vi "Sol_Tierra_Luna_2.vi"() -> ()   [LabVIEW 2016]
panel:
  out "Luna":bool
  in  "Posición Horizontal":i32(slide) scale=0.0..100.0
  in  "Posición Vertical":i32(slide) scale=0.0..100.0
  in  "Stop Button":bool
  out "Tierra":bool
  out "Sol":bool
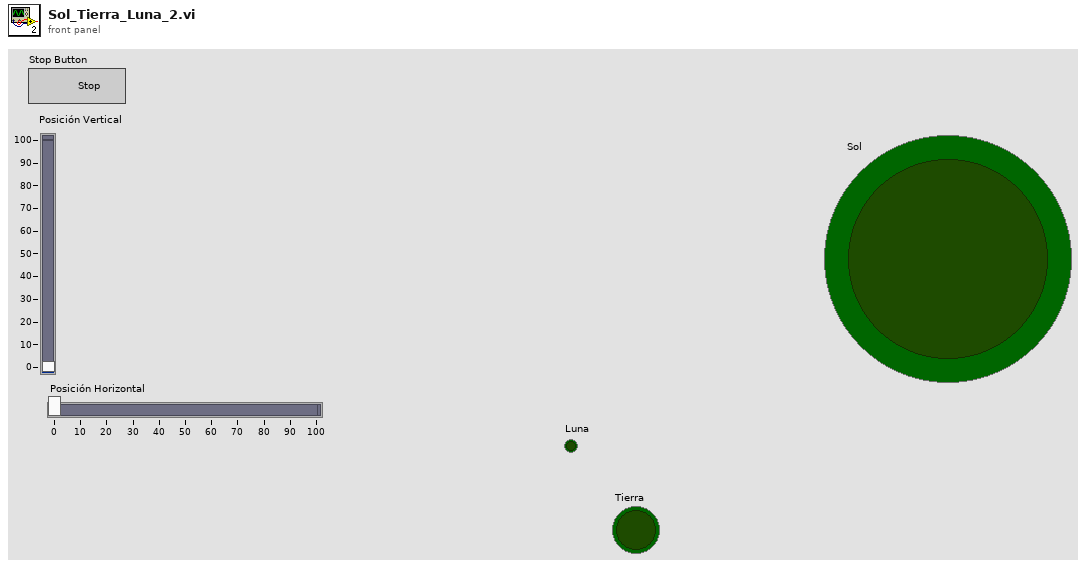
[diagram p1: front panel]
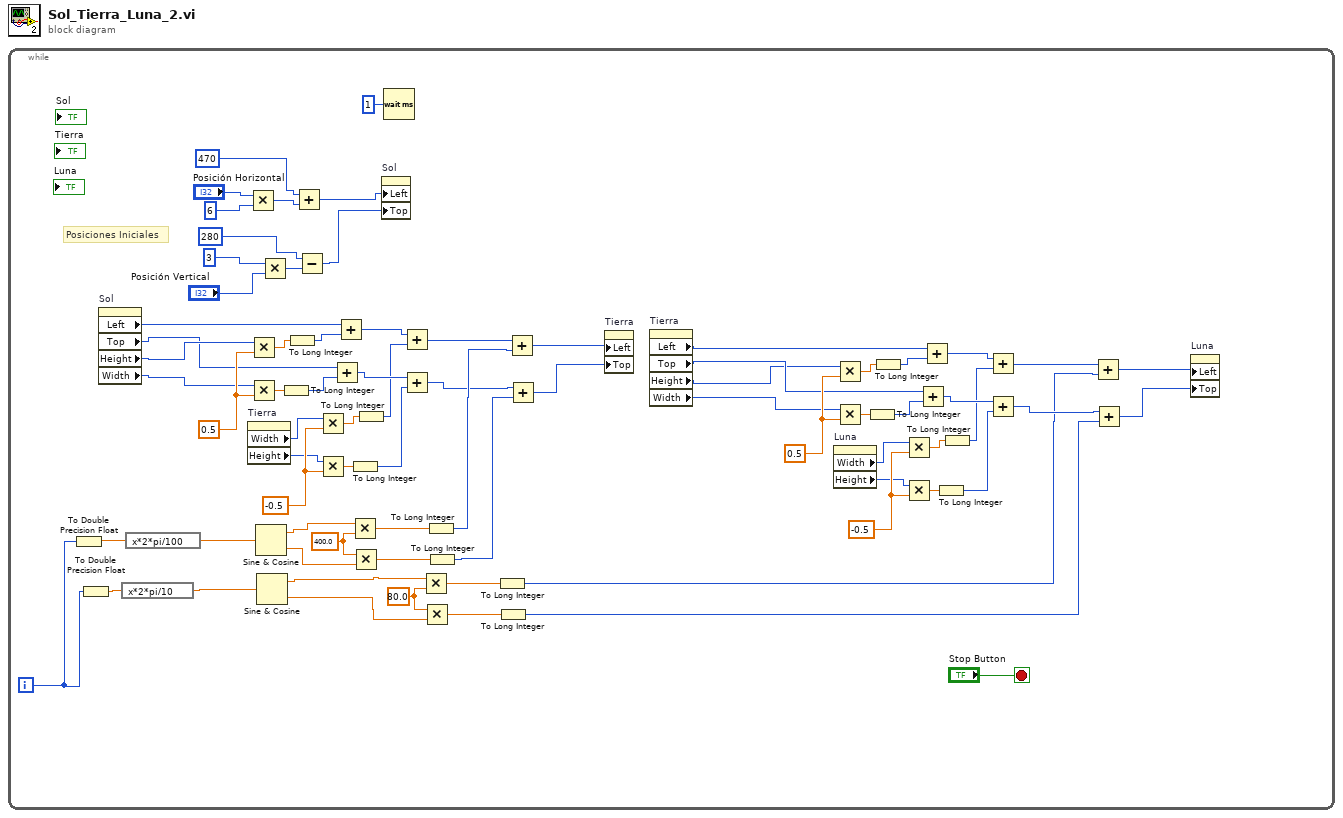
[diagram p0: block diagram]
diagram:
  n1 = while {
    i -> [w40]
    stop <- "Stop Button" stop-if-true
    w17 = -0.5 ("y")
    w20 = 0.5 ("y")
    w29 = 80.0 ("y")
    w38 = 400.0 ("y")
    w62 = -0.5 ("y")
    w69 = 0.5 ("y")
    # "Posiciones Iniciales"
    n2 = To Double Precision Float(number=w40) -> (double precision float=w41:dbl)
    n3 = To Double Precision Float(number=w40) -> (double precision float=w43:dbl)
    n4 = property on="Sol" class="Bool (strict)"() -> ("Left"=w65:i32, "Top"=w66:i32, "Height"=w67:u32, "Width"=w68:u32)  [unwired: 2 in, 2 out]
    n5 = expression code="x*2*pi/10"(w43) -> (w45:dbl)
    n6 = expression code="x*2*pi/100"(w41) -> (w44:dbl)
    n7 = Multiply(x="Posición Horizontal", y=6) -> (x*y=w48:i32)
    n8 = property on="Tierra" class="Bool (strict)"() -> ("Width"=w61:u32, "Height"=w60:u32)  [unwired: 2 in, 2 out]
    n9 = Multiply(x=w67, y=w69) -> (x*y=w71:dbl)
    n10 = Multiply(x=w68, y=w69) -> (x*y=w73:dbl)
    n11 = Sine & Cosine(0:w44) -> (1:w39:dbl, 2:w42:dbl)
    n12 = Sine & Cosine(0:w45) -> (1:w26:dbl, 2:w25:dbl)
    n13 = Multiply(x=3, y="Posición Vertical") -> (x*y=w55:i32)
    n14 = To Long Integer(number=w73) -> (32bit integer=w72:i32)
    n15 = To Long Integer(number=w71) -> (32bit integer=w70:i32)
    n16 = Add(x=470 ("Position:Left"), y=w48) -> (x+y=w47:i32)
    n17 = Subtract(x=280 ("Position:Top"), y=w55) -> (x-y=w46:i32)
    n18 = Multiply(x=w61, y=w62) -> (x*y=w63:dbl)
    n19 = Multiply(x=w60, y=w62) -> (x*y=w64:dbl)
    n20 = Add(x=w66, y=w72) -> (x+y=w59:i32)
    n21 = Add(x=w65, y=w70) -> (x+y=w58:i32)
    n22 = To Long Integer(number=w64) -> (32bit integer=w56:i32)
    n23 = Multiply(x=w39, y=w38) -> (x*y=w36:dbl)
    n24 = Multiply(x=w38, y=w42) -> (x*y=w37:dbl)
    n25 = To Long Integer(number=w63) -> (32bit integer=w57:i32)
    n26 = property on="Sol" class="Bool (strict)"("Left"=w47, "Top"=w46) -> ()  [unwired: 2 in, 2 out]
    n27 = Wait (ms)(milliseconds to wait=u32 1) -> ()  [unwired: 1 out]
    n28 = Add(x=w58, y=w57) -> (x+y=w32:i32)
    n29 = Add(x=w59, y=w56) -> (x+y=w33:i32)
    n30 = Multiply(x=w26, y=w29) -> (x*y=w27:dbl)
    n31 = Multiply(x=w29, y=w25) -> (x*y=w28:dbl)
    n32 = To Long Integer(number=w36) -> (32bit integer=w35:i32)
    n33 = To Long Integer(number=w37) -> (32bit integer=w34:i32)
    n34 = To Long Integer(number=w27) -> (32bit integer=w4:i32)
    n35 = To Long Integer(number=w28) -> (32bit integer=w3:i32)
    n36 = Add(x=w32, y=w35) -> (x+y=w31:i32)
    n37 = Add(x=w33, y=w34) -> (x+y=w30:i32)
    n38 = property on="Tierra" class="Bool (strict)"("Left"=w31, "Top"=w30) -> ()  [unwired: 2 in, 2 out]
    n39 = property on="Tierra" class="Bool (strict)"() -> ("Left"=w8:i32, "Top"=w7:i32, "Height"=w6:u32, "Width"=w5:u32)  [unwired: 2 in, 2 out]
    n40 = property on="Luna" class="Bool (strict)"() -> ("Width"=w16:u32, "Height"=w15:u32)  [unwired: 2 in, 2 out]
    n41 = Multiply(x=w6, y=w20) -> (x*y=w22:dbl)
    n42 = Multiply(x=w5, y=w20) -> (x*y=w24:dbl)
    n43 = To Long Integer(number=w24) -> (32bit integer=w23:i32)
    n44 = To Long Integer(number=w22) -> (32bit integer=w21:i32)
    n45 = Multiply(x=w16, y=w17) -> (x*y=w18:dbl)
    n46 = Multiply(x=w15, y=w17) -> (x*y=w19:dbl)
    n47 = Add(x=w7, y=w23) -> (x+y=w14:i32)
    n48 = Add(x=w8, y=w21) -> (x+y=w13:i32)
    n49 = To Long Integer(number=w19) -> (32bit integer=w11:i32)
    n50 = To Long Integer(number=w18) -> (32bit integer=w12:i32)
    n51 = Add(x=w13, y=w12) -> (x+y=w9:i32)
    n52 = Add(x=w14, y=w11) -> (x+y=w10:i32)
    n53 = Add(x=w9, y=w4) -> (x+y=w1:i32)
    n54 = Add(x=w10, y=w3) -> (x+y=w2:i32)
    n55 = property on="Luna" class="Bool (strict)"("Left"=w1, "Top"=w2) -> ()  [unwired: 2 in, 2 out]
  }
